vi "Motors Speed.vi"() -> ()   [LabVIEW 2016]
panel:
  in  "Measured motor speed rev/s":dbl
  in  "Measured Left motor speed rev/s":dbl
  in  "Right motor speed rev/s":dbl
  in  "Left motor speed rev/s":dbl
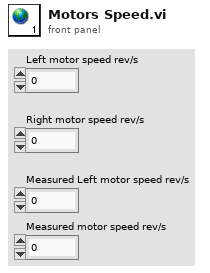
[diagram p1: front panel]
diagram:
